vi "Create gRPC Client.vi"(8 "error in (no error)":errorcluster, 11 "FlexLogger_gRPC in":refnum<class "FlexLogger_gRPC.lvclass">) -> (0 "error out":errorcluster, 3 "FlexLogger_gRPC out":refnum<class "FlexLogger_gRPC.lvclass">)   [LabVIEW 2020, in "FlexLogger_gRPC.lvlib" / "FlexLogger_gRPC.lvclass"]
uses:
  FlexLogger_gRPC.lvclass
  FlexLogger_gRPC.lvclass/FlexLogger_gRPC.ctl
  FlexLogger_client/FlexLogger_client.lvlib
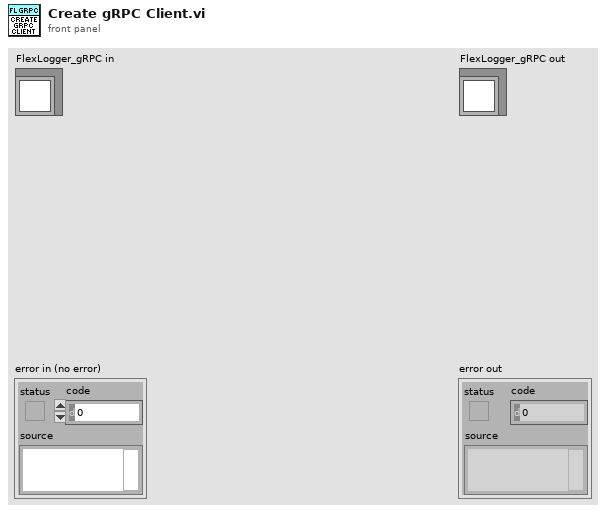
[diagram p1: front panel]
types:
  T1 = typedef "grpc-lvsupport-release.lvlib/grpcId.ctl" = u64
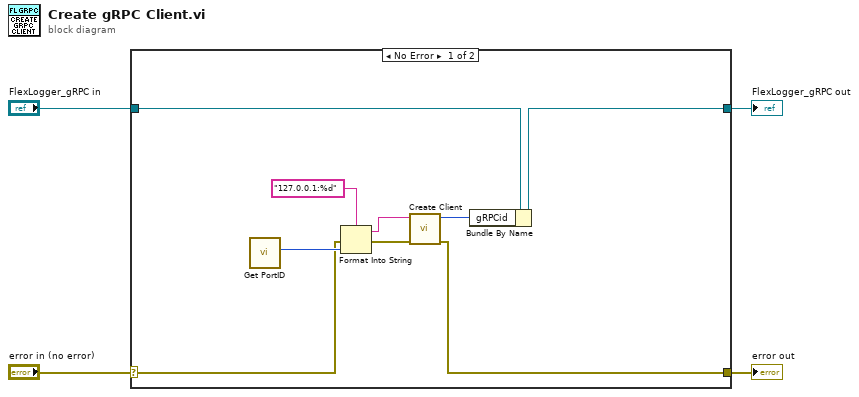
[diagram p0: block diagram]
diagram:
  n1 = case shown="No Error" "error in (no error)" {
    selector: "error in (no error)" -> [w6 w15]
    tunnel: [w13 w15] -> w3
    tunnel: [w11 w14] -> w1
    tunnel: "FlexLogger_gRPC in" -> [w10 w14]
    frame No Error {
      n2 = call "Get PortID.vi"() -> ("PortID"=w9:i32)  [unwired: 11 in]
      n3 = Format Into String(format string="127.0.0.1:%d" ("address"), error in=w6, w9) -> (resulting string=w7:string, error out=w5:errorcluster)  [unwired: 1 in]
      n4 = call "Create Client.vi"("error in"=w5, "address"=w7) -> ("error out"=w13:errorcluster, "gRPC ID Out"=w12:T1)  [unwired: 8 in]
      n5 = Bundle By Name(cluster=w10, "gRPCid"=w12) -> (w11:refnum<class "FlexLogger_gRPC.lvclass">)
    }
    frame Error {
    }
  }
  "error out" <- w3
  "FlexLogger_gRPC out" <- w1
